vi "MIDI_Error_Check.vi"(8 "error in (no error)":errorcluster, 11 "Numeric":i32) -> (0 "error out":errorcluster)   [LabVIEW 2019]
uses:
  winmm.dll
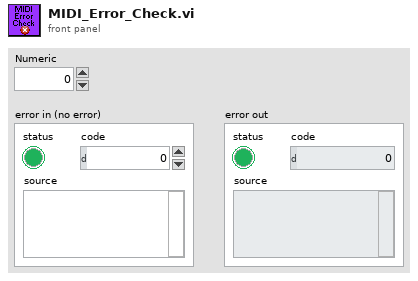
[diagram p1: front panel]
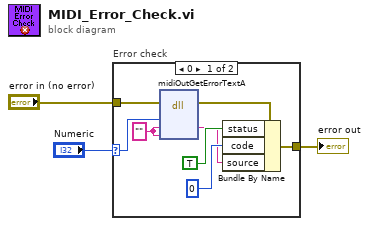
[diagram p0: block diagram]
diagram:
  n1 = case "Error check" shown="0" "Numeric" {
    selector: "Numeric" -> [w11 _]
    tunnel: "error in (no error)" -> [w10 w12]
    tunnel: [w7 w12] -> w2
    frame 0 {
      w9 = "" ("pszText")
      n2 = dll-call lib="winmm.dll" fn="midiOutGetErrorTextA"(error in=w10, "mmrError"=w11, "pszText"=w9, "cchText"=w9) -> (error out=w8:errorcluster, "pszText"=w4:string)  [unwired: 5 in, 1 out]
      n3 = Bundle By Name(cluster=w8, "status"=TRUE, "code"=0, "source"=w4) -> (w7:errorcluster)
    }
    frame 1.., Default {
    }
  }
  "error out" <- w2
